vi "Make Counter Signal If Match.vi"(5 "Counter Value GUID":string="94e87467-031b-484c-a85e-bcbac581524d", 7 "Protected Signal GUID":string="D95BE1B9-793B-430A-998F-7F352C03EC7C", 8 "error in (no error)":errorcluster, 10 "Cluster":cluster{"Name":string, "Item Ref out":T1} {"Item Ref out" format="%.0x"}, 11 "Matching Strings":string[](array[string])) -> (0 "error out":errorcluster)   [LabVIEW 2023, in "Protection and Counter Support System Explorer.lvlib"]
uses:
  Protection and Counter Support System Explorer.lvlib
  <vilib>/NI VeriStand/Custom Device API/Custom Device Item Ref.ctl
  <vilib>/NI VeriStand/Custom Device API/Custom Device API.lvlib
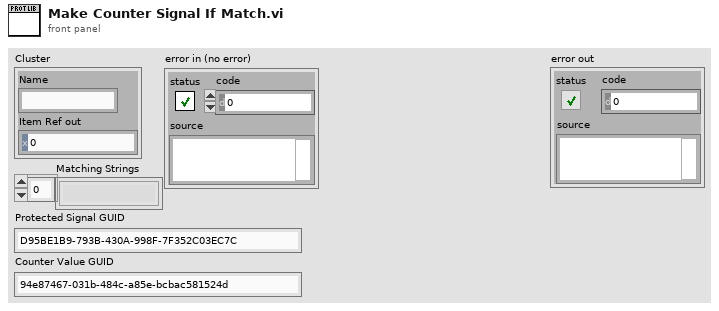
[diagram p1: front panel]
types:
  T1 = typedef "Custom Device API.lvlib/Custom Device Item Ref.ctl" = u64
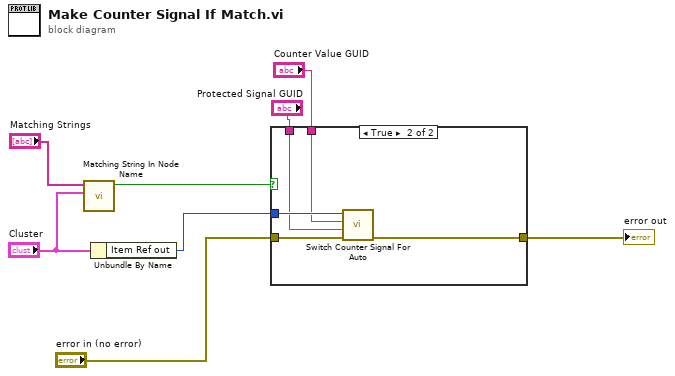
[diagram p0: block diagram]
diagram:
  n1 = call "Matching String In Node Name.vi"("Cluster"="Cluster", "Matching Strings"="Matching Strings") -> ("found?"=w7:bool)  [unwired: 9 in]
  n2 = Unbundle By Name("Cluster") -> ("Item Ref out"=w5:T1)
  n3 = case shown="True" w7 {
    tunnel: w5 -> [_ w14]
    tunnel: [w9 w13] -> w4
    tunnel: "error in (no error)" -> [w9 w12]
    tunnel: "Counter Value GUID" -> [_ w11]
    tunnel: "Protected Signal GUID" -> [_ w10]
    frame False {
    }
    frame True {
      n4 = call "Switch Counter Signal For Auto.vi"("error in (no error)"=w12, "Protected Signal GUID"=w10, "Counter Value GUID"=w11, "Node Ptr"=w14) -> ("error out"=w13:errorcluster)  [unwired: 7 in]
    }
  }
  "error out" <- w4
